vi "Rectangle%.vi"(10 "Rectangle Array ltrb":dbl[](array[numeric])=[2.22, 1.4], 11 "Convex Hull Area":dbl) -> (3 "Score":dbl)   [LabVIEW 2017]
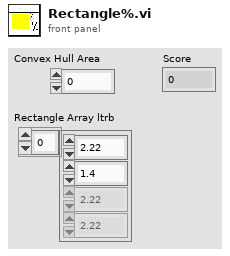
[diagram p1: front panel]
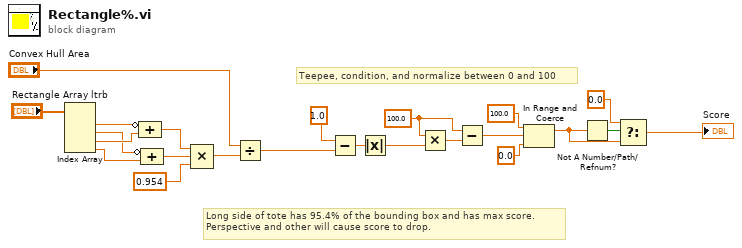
[diagram p0: block diagram]
diagram:
  w16 = 100.0 ("x/y")
  # "Teepee, condition, and normalize between 0 and 100"
  # "Long side of tote has 95.4% of the bounding box and has max score.\nPerspective and other will cause score to drop."
  n1 = Index Array(array="Rectangle Array ltrb") -> (element #1=w7:dbl, element #2=w4:dbl, element #3=w6:dbl, element #4=w5:dbl)  [unwired: 4 in]
  n2 = Compound Arithmetic op=ADD(invert w7, w6) -> (w9:dbl)
  n3 = Compound Arithmetic op=ADD(invert w4, w5) -> (w10:dbl)
  n4 = Compound Arithmetic op=MULTIPLY(w9, w10, 0.954 ("y")) -> (w3:dbl)
  n5 = Divide(x="Convex Hull Area", y=w3) -> (x/y=w19:dbl)
  n6 = Subtract(x=1.0 ("y"), y=w19) -> (x-y=w14:dbl)
  n7 = Absolute Value(x=w14) -> (abs(x)=w17:dbl)
  n8 = Multiply(x=w16, y=w17) -> (x*y=w18:dbl)
  n9 = Subtract(x=w16, y=w18) -> (x-y=w13:dbl)
  n10 = In Range and Coerce(upper limit=100.0, x=w13, lower limit=0.0) -> (coerced(x)=w22:dbl)  [unwired: 1 out]
  n11 = Not A Number/Path/Refnum?(number/path/refnum=w22) -> (NaN/Path/Refnum?=w21:bool)
  n12 = Select(t=0.0 ("y"), s=w21, f=w22) -> (s? t:f=→"Score":dbl)
